vi "Find Subaddress.vi"(8 "error in":errorcluster, 10 "subaddress":T1, 11 "remote terminal":T2 format="%.0x") -> (0 "error out":errorcluster, 2 "subaddress section":T2 format="%.0x", 3 "remote terminal out":T2 format="%.0x", 4 "found?":bool)   [LabVIEW 2020, in "AIM MIL-STD-1553 Scripting.lvlib"]
doc: "Returns a <b>subaddress section</b> that contains the specified <b>subaddress</b> value."
uses:
  AIM MIL-STD-1553 Scripting.lvlib
  <vilib>/NI VeriStand/Custom Device API/Custom Device Item Ref.ctl
  Shared/Address.ctl
  <vilib>/NI VeriStand/Custom Device API/Custom Device API.lvlib
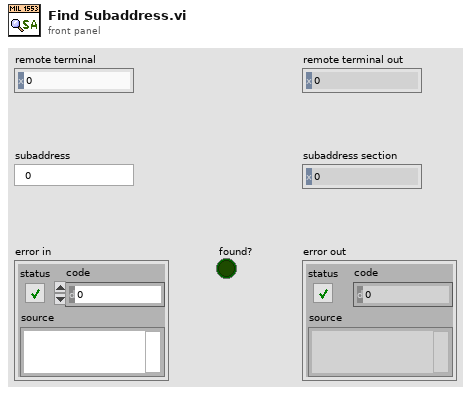
[diagram p1: front panel]
types:
  T1 = typedef "Address.ctl" = u16
  T2 = typedef "Custom Device API.lvlib/Custom Device Item Ref.ctl" = u64
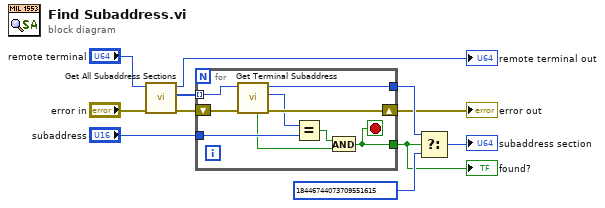
[diagram p0: block diagram]
diagram:
  n1 = call "Get All Subaddress Sections.vi"("error in"="error in", "remote terminal"="remote terminal") -> ("error out"=w6:errorcluster, "subaddress sections"=w3:T2[], "remote terminal out"=→"remote terminal out":T2)  [unwired: 7 in]
  n2 = for {
    tunnel: w3 -> [w20] mode=indexing
    tunnel: "subaddress" -> [w19]
    tunnel: [w14] -> w11
    tunnel: [w13] -> w2
    shift-right: [w15] -> w5
    shift-left: w6 -> [w16]
    stop <- w13 stop-if-true
    n3 = call "Get Terminal Subaddress.vi"("error in"=w16, "subaddress section"=w20) -> ("error out"=w15:errorcluster, "subaddress value"=w12:T1, "subaddress section out"=w14:T2, "found?"=w18:bool)  [unwired: 6 in]
    n4 = Equal?(x=w12, y=w19) -> (x = y?=w17:bool)
    n5 = And(x=w17, y=w18) -> (x .and. y?=w13:bool)
  }
  "error out" <- w5
  "found?" <- w2
  n6 = Select(t=w11, s=w2, f=T2 18446744073709551615 ("Invalid Ref")) -> (s? t:f=→"subaddress section":T2)
